vi "Make Grid Overlay.vi"(7 "Grid Size (10)":i32=10, 11 "Maze":refnum<class "Maze.lvclass">) -> (3 "Picture":picture)   [LabVIEW 2020, in "App.lvlib" / "MazeUI.lvclass"]
uses:
  MazeUI.lvclass
  build/ppl/maze.lvlibp/Maze/Maze.lvclass
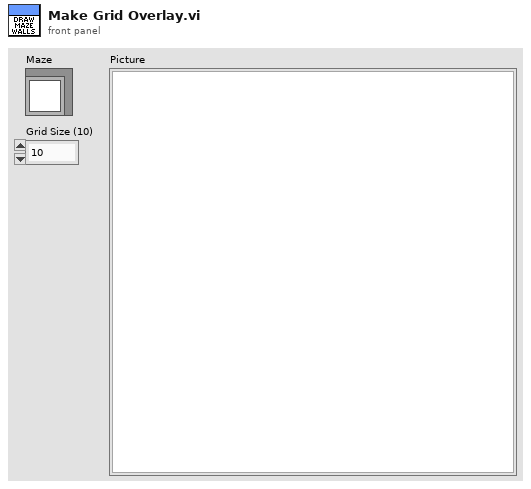
[diagram p1: front panel]
types:
  T1 = typedef "maze.lvlibp/Adjacency.ctl" = cluster{"E":bool, "N":bool, "W":bool, "S":bool, "Goal":bool, "Start":bool}
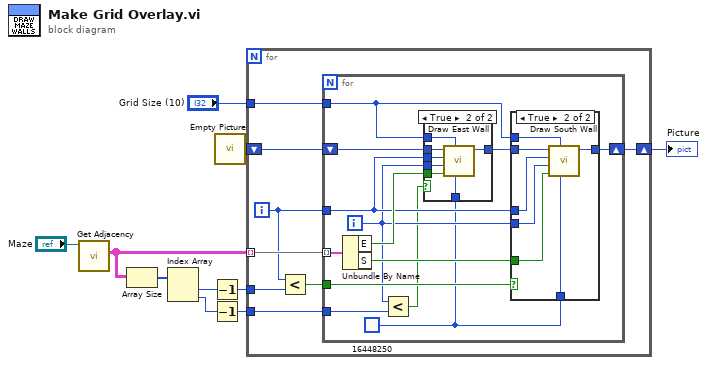
[diagram p0: block diagram]
diagram:
  n1 = call "Get Adjacency.vi"("Maze in"="Maze") -> ("Adjacency"=w8:T1[][])  [unwired: 8 in, 2 out]
  n2 = Array Size(array=w8) -> (size(s)=w9:i32[])
  n3 = Index Array(array=w9) -> (element #1=w6:i32, element #2=w4:i32)  [unwired: 2 in]
  n4 = Decrement(x=w6) -> (x-1=w5:i32)
  n5 = Decrement(x=w4) -> (x-1=w3:i32)
  n6 = call "Empty Picture"() -> ("empty picture"=w7:picture)
  n7 = for {
    tunnel: w8 -> [w18] mode=indexing
    shift-right: [w16] -> w2
    shift-left: w7 -> [w17]
    tunnel: w5 -> [w15]
    tunnel: w3 -> [w12]
    tunnel: "Grid Size (10)" -> [w11]
    i -> [w14]
    n8 = Less?(x=w14, y=w15) -> (x < y?=w13:bool)
    n9 = for {
      tunnel: w18 -> [w31] mode=indexing
      shift-right: [w24] -> w16
      shift-left: w17 -> [w30]
      tunnel: w14 -> [w26]
      tunnel: w13 -> [w28]
      tunnel: w12 -> [w23]
      tunnel: w11 -> [w19]
      i -> [w22]
      w20 = u32 16448250 ("color")
      n10 = Unbundle By Name(w31) -> ("E"=w29:bool, "S"=w27:bool)
      n11 = Less?(x=w22, y=w23) -> (x < y?=w21:bool)
      n12 = case shown="True" w21 {
        tunnel: w30 -> [w32 w39]
        tunnel: w29 -> [_ w38]
        tunnel: w26 -> [_ w37]
        tunnel: [w32 w36] -> w25
        tunnel: w22 -> [_ w35]
        tunnel: w20 -> [_ w34]
        tunnel: w19 -> [_ w33]
        frame False {
        }
        frame True {
          n13 = call "Draw East Wall.vi"("color"=w34, "Grid Size (10)"=w33, "Connected"=w38, "Col"=w35, "Row"=w37, "Picture In"=w39) -> ("Picture"=w36:picture)  [unwired: 5 in]
        }
      }
      n14 = case shown="True" w28 {
        tunnel: w27 -> [_ w43]
        tunnel: w26 -> [_ w45]
        tunnel: w22 -> [_ w44]
        tunnel: w25 -> [w40 w47]
        tunnel: [w40 w46] -> w24
        tunnel: w20 -> [_ w42]
        tunnel: w19 -> [_ w41]
        frame False {
        }
        frame True {
          n15 = call "Draw South Wall.vi"("color"=w42, "Grid Size (10)"=w41, "Connected"=w43, "Col"=w44, "Row"=w45, "Picture In"=w47) -> ("Picture"=w46:picture)  [unwired: 5 in]
        }
      }
    }
  }
  "Picture" <- w2
